vi "Head and Tail Detection (SubVI).vi"(0 "Boundary Point XY":u32, 1 "Bondary Valid?":bool, 2 "Scan End?":bool, 6 "Significant Angle":fxp<+,16,3>=0.0999755859375 format="%#_14g", 8 "Min Contour Points":u16=63) -> (11 "Ready for Input?":bool, 14 "Output Valid?":bool, 15 "Skip Contour Analysis":bool, 17 "V1 Index":u16, 18 "V2 Index":u16, 19 "N Points":u16)   [LabVIEW 2015]
uses:
  Controls (FPGA)/Head Tail Detection.ctl
  <vilib>/rvi/Memory/Memory_Emulation/nirvimemoryFastEmulation.vi
  <vilib>/rvi/Memory/Memory_Emulation/nirvimemoryEmulation.vi
  <vilib>/rvi/Emulation/niFpgaEmulationIsFPGAContextNoSignature.vi
  <vilib>/rvi/DataTransferAndStorage/Container/Common/niFpgaContainerGetUniqueNameForEmu.vi
  <vilib>/rvi/Emulation/niFpgaProcessEmulError.vi
  <vilib>/rvi/Emulation/niFpgaSctlEmulationGetInTimedLoop.vi
  <vilib>/rvi/errors/nirviReportUnexpectedCaseInternalError (U32).vi
  <vilib>/rvi/interface/RandomDataEmulation/niFpgaRandomDataHandleErrors.vi
  <vilib>/rvi/DataTransferAndStorage/Container/XNode/niFpgaContainer.xnode
  <vilib>/rvi/interface/RandomDataEmulation/nirviRandomDataFpgaReadWriteTemplate.vi
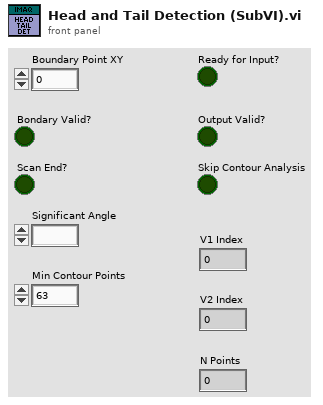
[diagram p1: front panel]
types:
  T1 = typedef "Head Tail Detection.ctl" = enum16{"Receive Contour Points", "Compute Angle", "Find Head", "Find Tail Search Region", "Find Tail"}
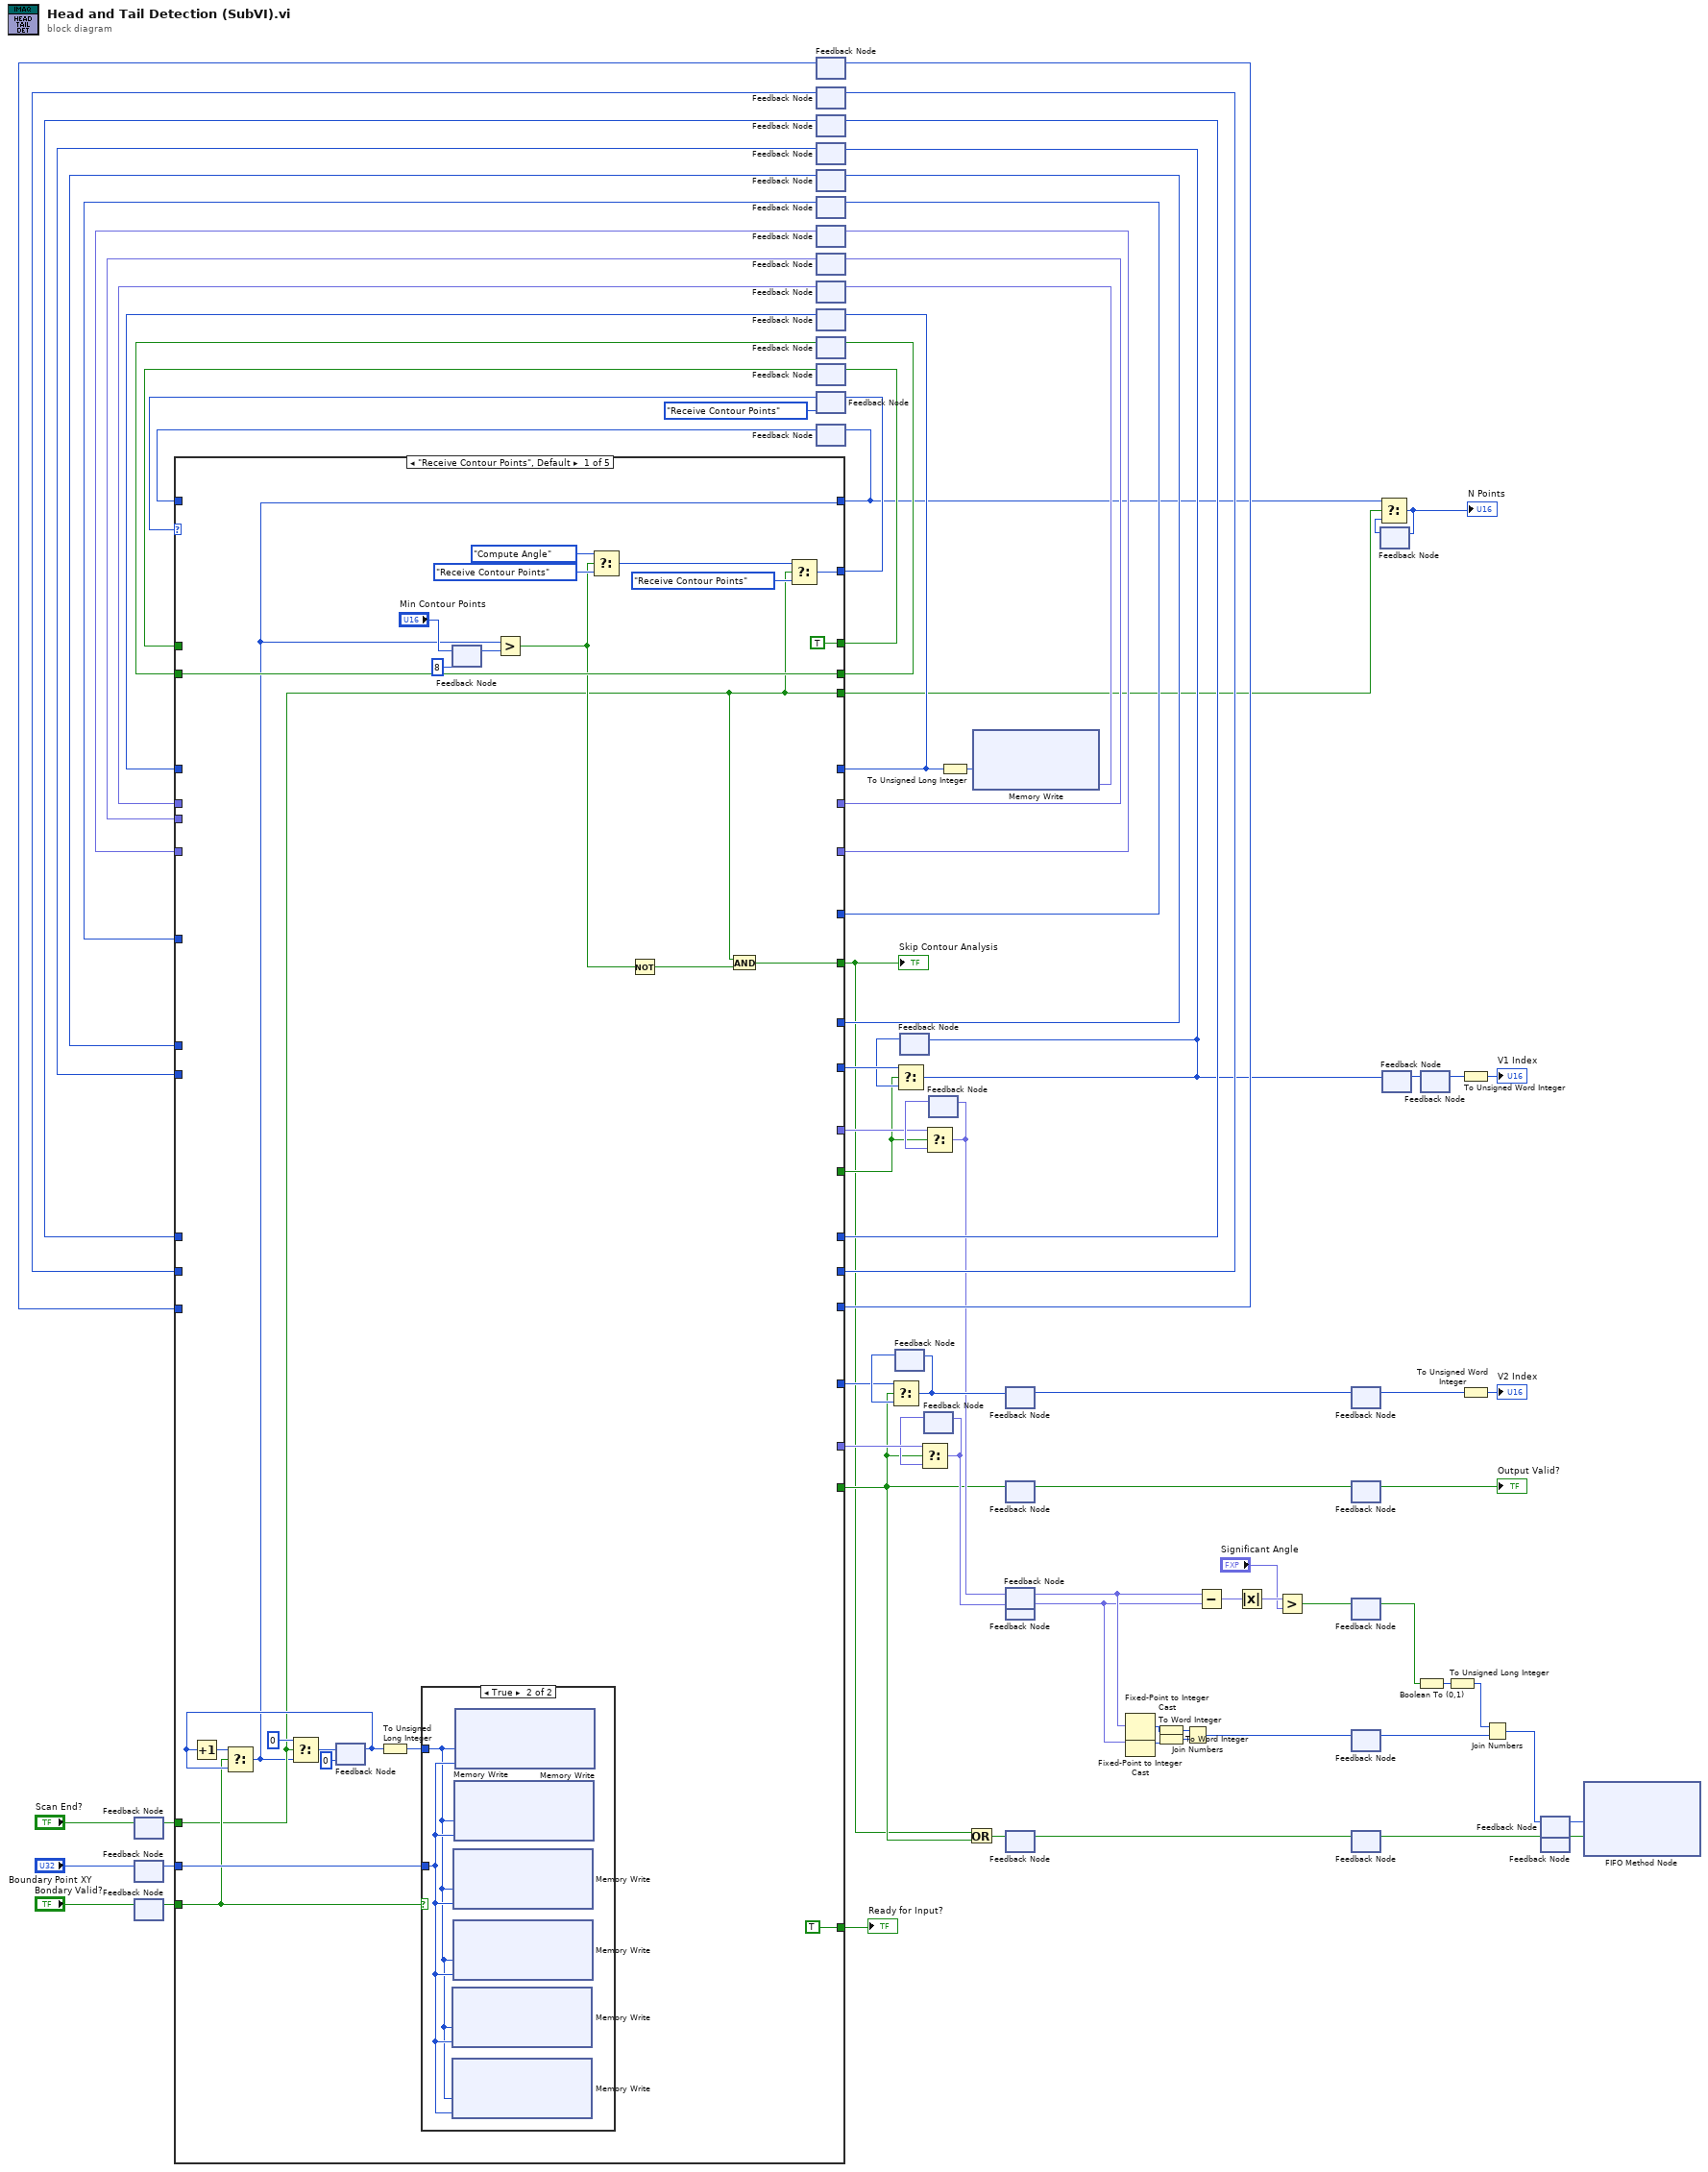
[diagram p0: block diagram]
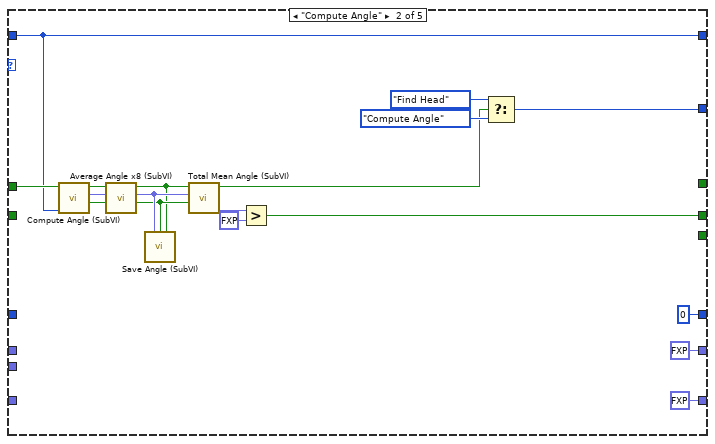
[diagram p3: hidden frame]
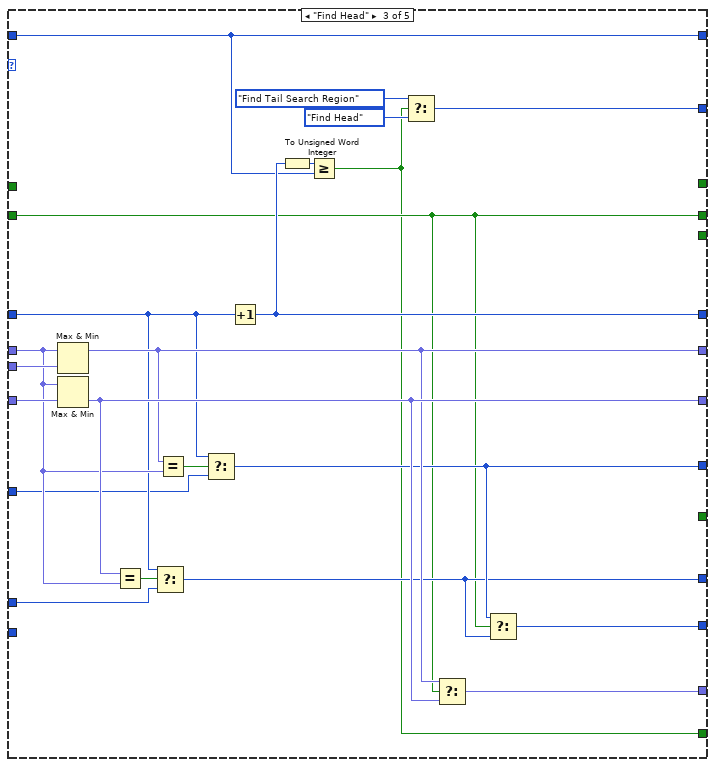
[diagram p4: hidden frame]
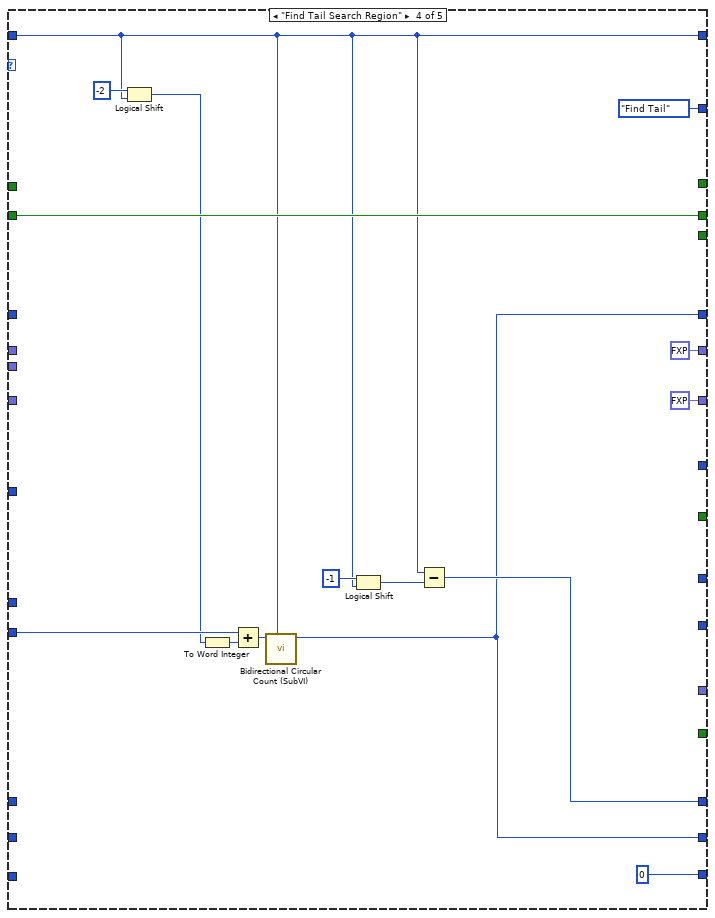
[diagram p5: hidden frame]
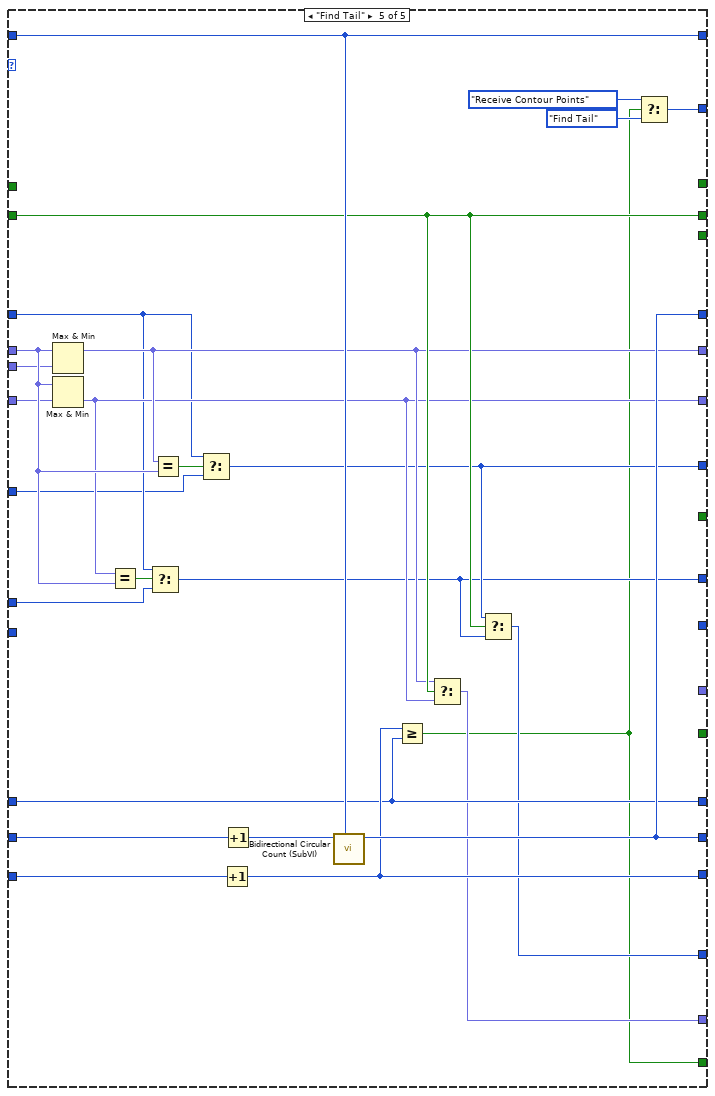
[diagram p6: hidden frame]
diagram:
  n1 = feedback-in #1("Scan End?") -> ()
  n2 = feedback #1() -> (w71:bool)  [unwired: 1 in]
  n3 = feedback-in #2("Boundary Point XY") -> ()
  n4 = feedback #2() -> (w72:u32)  [unwired: 1 in]
  n5 = feedback-in #3("Bondary Valid?") -> ()
  n6 = feedback #3() -> (w80:bool)  [unwired: 1 in]
  n7 = feedback #4() -> (w39:u16)  [unwired: 1 in]
  n8 = feedback #5() -> (w41:i16)  [unwired: 1 in]
  n9 = feedback #6() -> (w43:u16)  [unwired: 1 in]
  n10 = feedback #7() -> (w45:i16)  [unwired: 1 in]
  n11 = feedback #8() -> (w51:i16)  [unwired: 1 in]
  n12 = feedback #9() -> (w53:i16)  [unwired: 1 in]
  n13 = feedback #10() -> (w55:fxp<+/-,16,3>)  [unwired: 1 in]
  n14 = feedback #11() -> (w57:fxp<+/-,16,3>)  [unwired: 1 in]
  n15 = feedback #12() -> (w59:fxp<+/-,16,3>)  [unwired: 1 in]
  n16 = feedback #13() -> (w63:i16)  [unwired: 1 in]
  n17 = feedback #14() -> (w64:bool)  [unwired: 1 in]
  n18 = feedback #15() -> (w66:bool)  [unwired: 1 in]
  n19 = feedback #16(Head_Tail_Detection."Receive Contour Points") -> (w73:T1)
  n20 = feedback #17() -> (w69:u16)  [unwired: 1 in]
  n21 = case shown="\"Receive Contour Points\", Default" w73 {
    tunnel: w72 -> [w106 _ _ _ _]
    tunnel: w80 -> [w95 _ _ _ _]
    tunnel: w71 -> [w87 _ _ _ _]
    tunnel: [w102 w126 w146 Head_Tail_Detection."Find Tail" w188] -> w70
    tunnel: [w86 w117 w144 w156 w184] -> w23
    tunnel: w69 -> [_ w117 w144 w156 w184]
    tunnel: [TRUE _ _ _ _] -> w68
    tunnel: [TRUE _ _ _ _] -> w67
    tunnel: w66 -> [_ w119 _ _ _]
    tunnel: [w92 w114 w130 w164 w178] -> w65
    tunnel: w64 -> [w92 _ w130 w164 w178]
    tunnel: [_ i16 0 ("Count Out") w145 w152 w183] -> w61
    tunnel: w63 -> [_ _ w136 _ w172]
    tunnel: w59 -> [_ _ w137 _ w177]
    tunnel: [_ fxp<+/-,16,3> 0.0 w138 fxp<+/-,16,3> 0.0 w174] -> w58
    tunnel: [_ fxp<+/-,16,3> 2.0 w141 fxp<+/-,16,3> 2.0 w173] -> w56
    tunnel: w57 -> [_ _ w149 _ w176]
    tunnel: w55 -> [_ _ w142 _ w175]
    tunnel: [_ _ w131 _ w168] -> w52
    tunnel: [_ _ w132 _ w169] -> w54
    tunnel: w53 -> [_ _ w135 _ w171]
    tunnel: w51 -> [_ _ w134 _ w170]
    tunnel: [_ _ w133 _ _] -> w47
    tunnel: [_ _ w129 _ _] -> w50
    tunnel: [_ _ w128 _ _] -> w46
    tunnel: w45 -> [_ _ _ w161 _]
    tunnel: [_ _ _ w152 w183] -> w42
    tunnel: [_ _ _ w154 w181] -> w44
    tunnel: w43 -> [_ _ _ _ w181]
    tunnel: w41 -> [_ _ _ _ w186]
    tunnel: [w88 _ _ _ _] -> w11
    tunnel: [_ _ _ u16 0 ("x-y") w182] -> w40
    tunnel: w39 -> [_ _ _ _ w187]
    tunnel: [_ _ _ _ w166] -> w38
    tunnel: [_ _ _ _ w167] -> w35
    tunnel: [_ _ _ _ w165] -> w18
    tunnel: [w87 _ _ _ _] -> w20
    frame "Receive Contour Points", Default {
      n22 = feedback #18(u16 0 ("Count")) -> (w96:u16)
      n23 = Increment(x=w96) -> (x+1=w97:u16)
      n24 = Select(t=w97, s=w95, f=w96) -> (s? t:f=w86:u16)
      n25 = Select(t=u16 0 ("Count"), s=w87, f=w86) -> (s? t:f=w89:u16)
      n26 = feedback-in #18(w89) -> ()
      n27 = To Unsigned Long Integer(number=w96) -> (unsigned 32bit integer=w107:u32)
      n28 = case shown="True" w95 {
        tunnel: w106 -> [_ w109]
        tunnel: w107 -> [_ w108]
        frame False {
        }
        frame True {
          n29 = xnode ("Memory Write")("Address"=w108, "Data"=w109) -> ()  [unwired: 1 in, 1 out]
          n30 = xnode ("Memory Write")("Address"=w108, "Data"=w109) -> ()  [unwired: 1 in, 1 out]
          n31 = xnode ("Memory Write")("Address"=w108, "Data"=w109) -> ()  [unwired: 1 in, 1 out]
          n32 = xnode ("Memory Write")("Address"=w108, "Data"=w109) -> ()  [unwired: 1 in, 1 out]
          n33 = xnode ("Memory Write")("Address"=w108, "Data"=w109) -> ()  [unwired: 1 in, 1 out]
          n34 = xnode ("Memory Write")("Address"=w108, "Data"=w109) -> ()  [unwired: 1 in, 1 out]
        }
      }
      n35 = feedback-in #19("Min Contour Points") -> ()
      n36 = feedback #19(u16 8 ("y")) -> (w85:u16)
      n37 = Greater?(x=w86, y=w85) -> (0:w91:bool)
      n38 = Select(t=Head_Tail_Detection."Compute Angle", s=w91, f=Head_Tail_Detection."Receive Contour Points") -> (s? t:f=w100:T1)
      n39 = Not(x=w91) -> (.not. x?=w90:bool)
      n40 = And(x=w87, y=w90) -> (x .and. y?=w88:bool)
      n41 = Select(t=w100, s=w87, f=Head_Tail_Detection."Receive Contour Points") -> (s? t:f=w102:T1)
    }
    frame "Compute Angle" {
      n42 = call "Compute Angle (SubVI).vi"("N Points"=w117, "Start"=w119) -> ("Angle Valid?"=w122:bool, "Angle"=w121:fxp<+/-,16,3>, "Done?"=w120:bool)  [unwired: 7 in]
      n43 = call "Average Angle x8 (SubVI).vi"("In Valid?"=w122, "Angle In"=w121, "End?"=w120) -> ("Out Valid?"=w124:bool, "Angle Out"=w125:fxp<+/-,16,3>, "Done?"=w123:bool)  [unwired: 6 in]
      n44 = call "Save Angle (SubVI).vi"("Angle"=w125, "In Valid?"=w124, "Done?"=w123) -> ()  [unwired: 13 in]
      n45 = call "Total Mean Angle (SubVI).vi"("Angle Valid"=w124, "Angle"=w125, "Done In"=w123) -> ("Mean Angle"=w116:fxp<+/-,32,16>, "Done Out"=w118:bool)  [unwired: 7 in]
      n46 = Greater?(x=w116, y=fxp<+/-,32,16> 1.0) -> (0:w114:bool)
      n47 = Select(t=Head_Tail_Detection."Find Head", s=w118, f=Head_Tail_Detection."Compute Angle") -> (s? t:f=w126:T1)
    }
    frame "Find Head" {
      n48 = Max & Min(x=w137, y=w149) -> (max(x,y)=w138:fxp<+/-,16,3>)  [unwired: 1 out]
      n49 = Max & Min(x=w137, y=w142) -> (min(x,y)=w141:fxp<+/-,16,3>)  [unwired: 1 out]
      n50 = Equal?(x=w141, y=w137) -> (x = y?=w140:bool)
      n51 = Select(t=w136, s=w140, f=w134) -> (s? t:f=w131:i16)
      n52 = Equal?(x=w138, y=w137) -> (x = y?=w139:bool)
      n53 = Select(t=w136, s=w139, f=w135) -> (s? t:f=w132:i16)
      n54 = Increment(x=w136) -> (x+1=w145:i16)
      n55 = To Unsigned Word Integer(number=w145) -> (unsigned 16bit integer=w143:u16)
      n56 = Greater Or Equal?(x=w143, y=w144) -> (x >= y?=w128:bool)
      n57 = Select(t=Head_Tail_Detection."Find Tail Search Region", s=w128, f=Head_Tail_Detection."Find Head") -> (s? t:f=w146:T1)
      n58 = Select(t=w138, s=w130, f=w141) -> (s? t:f=w133:fxp<+/-,16,3>)
      n59 = Select(t=w132, s=w130, f=w131) -> (s? t:f=w129:i16)
    }
    frame "Find Tail Search Region" {
      n60 = Logical Shift(y=i16 -2, x=w156) -> (x << y=w160:u16)
      n61 = To Word Integer(number=w160) -> (16bit integer=w159:i16)
      n62 = Add(x=w161, y=w159) -> (x+y=w158:i16)
      n63 = call "Bidirectional Circular Count (SubVI).vi"("Max. Count"=w156, "Count In"=w158) -> ("Count Out"=w152:i16)  [unwired: 9 in]
      n64 = Logical Shift(y=i16 -1, x=w156) -> (x << y=w155:u16)
      n65 = Subtract(x=w156, y=w155) -> (x-y=w154:u16)
    }
    frame "Find Tail" {
      n66 = Max & Min(x=w177, y=w176) -> (max(x,y)=w174:fxp<+/-,16,3>)  [unwired: 1 out]
      n67 = Max & Min(x=w177, y=w175) -> (min(x,y)=w173:fxp<+/-,16,3>)  [unwired: 1 out]
      n68 = Equal?(x=w173, y=w177) -> (x = y?=w180:bool)
      n69 = Select(t=w172, s=w180, f=w170) -> (s? t:f=w168:i16)
      n70 = Equal?(x=w174, y=w177) -> (x = y?=w179:bool)
      n71 = Select(t=w172, s=w179, f=w171) -> (s? t:f=w169:i16)
      n72 = Increment(x=w187) -> (x+1=w182:u16)
      n73 = Increment(x=w186) -> (x+1=w185:i16)
      n74 = call "Bidirectional Circular Count (SubVI).vi"("Max. Count"=w184, "Count In"=w185) -> ("Count Out"=w183:i16)  [unwired: 9 in]
      n75 = Greater Or Equal?(x=w182, y=w181) -> (x >= y?=w165:bool)
      n76 = Select(t=w174, s=w178, f=w173) -> (s? t:f=w166:fxp<+/-,16,3>)
      n77 = Select(t=w169, s=w178, f=w168) -> (s? t:f=w167:i16)
      n78 = Select(t=Head_Tail_Detection."Receive Contour Points", s=w165, f=Head_Tail_Detection."Find Tail") -> (s? t:f=w188:T1)
    }
  }
  "Skip Contour Analysis" <- w11
  "Ready for Input?" <- w68
  n79 = feedback-in #4(w40) -> ()
  n80 = feedback-in #5(w42) -> ()
  n81 = feedback-in #6(w44) -> ()
  n82 = feedback-in #8(w52) -> ()
  n83 = feedback-in #9(w54) -> ()
  n84 = feedback-in #10(w56) -> ()
  n85 = feedback-in #11(w58) -> ()
  n86 = feedback-in #13(w61) -> ()
  n87 = feedback-in #14(w65) -> ()
  n88 = feedback-in #15(w67) -> ()
  n89 = feedback-in #16(w70) -> ()
  n90 = feedback-in #17(w23) -> ()
  n91 = feedback #20() -> (w36:i16)  [unwired: 1 in]
  n92 = Select(t=w35, s=w18, f=w36) -> (s? t:f=w30:i16)
  n93 = feedback-in #20(w30) -> ()
  n94 = feedback #21() -> (w49:i16)  [unwired: 1 in]
  n95 = Select(t=w50, s=w46, f=w49) -> (s? t:f=w34:i16)
  n96 = feedback-in #7(w34) -> ()
  n97 = feedback-in #21(w34) -> ()
  n98 = feedback #22() -> (w37:fxp<+/-,16,3>)  [unwired: 1 in]
  n99 = Select(t=w38, s=w18, f=w37) -> (s? t:f=w27:fxp<+/-,16,3>)
  n100 = feedback-in #22(w27) -> ()
  n101 = feedback #23() -> (w48:fxp<+/-,16,3>)  [unwired: 1 in]
  n102 = Select(t=w47, s=w46, f=w48) -> (s? t:f=w28:fxp<+/-,16,3>)
  n103 = feedback-in #23(w28) -> ()
  n104 = To Unsigned Long Integer(number=w61) -> (unsigned 32bit integer=w62:u32)
  n105 = Or(x=w11, y=w18) -> (x .or. y?=w12:bool)
  n106 = xnode ("Memory Write")("Address"=w62) -> ("Data"=w60:fxp<+/-,16,3>)  [unwired: 1 in, 1 out]
  n107 = feedback-in #12(w60) -> ()
  n108 = feedback #24() -> (w31:i16)  [unwired: 1 in]
  n109 = feedback-in #24(w30) -> ()
  n110 = feedback-in #25(w18) -> ()
  n111 = feedback #25() -> (w75:bool)  [unwired: 1 in]
  n112 = feedback #26() -> (w17:fxp<+/-,16,3>)  [unwired: 1 in]
  n113 = feedback-in #26(w28) -> ()
  n114 = feedback #27() -> (w16:fxp<+/-,16,3>)  [unwired: 1 in]
  n115 = feedback-in #27(w27) -> ()
  n116 = feedback-in #28(w12) -> ()
  n117 = feedback #28() -> (w8:bool)  [unwired: 1 in]
  n118 = Fixed-Point to Integer Cast(1:w17) -> (0:w15:i16)
  n119 = Fixed-Point to Integer Cast(1:w16) -> (0:w14:i16)
  n120 = To Word Integer(number=w15) -> (16bit integer=w10:i16)
  n121 = To Word Integer(number=w14) -> (16bit integer=w9:i16)
  n122 = Join Numbers(hi=w10, lo=w9) -> ((hi.lo)=w13:u32)
  n123 = Subtract(x=w17, y=w16) -> (x-y=w79:fxp<+/-,17,4>)
  n124 = Absolute Value(x=w79) -> (abs(x)=w78:fxp<+,16,3>)
  n125 = Greater?(x=w78, y="Significant Angle") -> (0:w76:bool)
  n126 = feedback-in #29(w31) -> ()
  n127 = feedback #29() -> (w25:i16)  [unwired: 1 in]
  n128 = feedback-in #30(w75) -> ()
  n129 = feedback #30() -> (→"Output Valid?":bool)  [unwired: 1 in]
  n130 = feedback-in #31(w76) -> ()
  n131 = feedback #31() -> (w7:bool)  [unwired: 1 in]
  n132 = feedback #32() -> (w4:u32)  [unwired: 1 in]
  n133 = feedback-in #32(w13) -> ()
  n134 = feedback #33() -> (w19:bool)  [unwired: 1 in]
  n135 = feedback-in #33(w8) -> ()
  n136 = feedback #34() -> (w22:u16)  [unwired: 1 in]
  n137 = Select(t=w23, s=w20, f=w22) -> (s? t:f=w21:u16)
  "N Points" <- w21
  n138 = feedback-in #34(w21) -> ()
  n139 = feedback-in #35(w34) -> ()
  n140 = feedback #35() -> (w33:i16)  [unwired: 1 in]
  n141 = Boolean To (0,1)(Boolean=w7) -> (0, 1=w6:i16)
  n142 = feedback-in #36(w33) -> ()
  n143 = feedback #36() -> (w26:i16)  [unwired: 1 in]
  n144 = To Unsigned Long Integer(number=w6) -> (unsigned 32bit integer=w5:u32)
  n145 = To Unsigned Word Integer(number=w26) -> (unsigned 16bit integer=→"V1 Index":u16)
  n146 = To Unsigned Word Integer(number=w25) -> (unsigned 16bit integer=→"V2 Index":u16)
  n147 = Join Numbers(hi=w5, lo=w4) -> ((hi.lo)=w3:u64)
  n148 = feedback-in #37(w3) -> ()
  n149 = feedback #37() -> (w2:u64)  [unwired: 1 in]
  n150 = feedback-in #38(w19) -> ()
  n151 = feedback #38() -> (w1:bool)  [unwired: 1 in]
  n152 = xnode ("FIFO Method Node")("Element"=w2, "Input Valid"=w1) -> ()  [unwired: 1 in, 2 out]
